vi "RFSG_Control.vi"(8 "error in (no error)":errorcluster, 10 "Device Resources":T1={"RFSG Resource in"="5646R", "RFSA Resource in"="5646R", "RFmx Resource in"=""}, 11 "Message_Queues":T2) -> (0 "error out":errorcluster)   [LabVIEW 2014]
uses:
  02_Controls/Message_Queues.ctl
  02_Controls/Message_Data_Ctl.ctl
  15_DataManagement/Device_Resources.ctl
  15_DataManagement/Config_RFSG.ctl
  <instrlib>/niRFSG/niRFSG.llb/niRFSG Signal Names.ctl
  <instrlib>/niRFSG/niRFSG.llb/niRFSG Signal Identifiers.ctl
  <instrlib>/niRFSG/niRFSG.llb/niRFSG Exported Signal Destinations.ctl
  15_DataManagement/Change_Parameters.ctl
  <vilib>/RF Toolkits/GSM-EDGE/niGSMEDGE.lvlib
panel:
  out "Message":string
  in  "WfmList":string[](array[string])=["LTE", "WCDMA", "GSM", "EDGE", "CW", "CWM"]
  out "RFSG Resource out":refnum<k15>="5644R (17)"
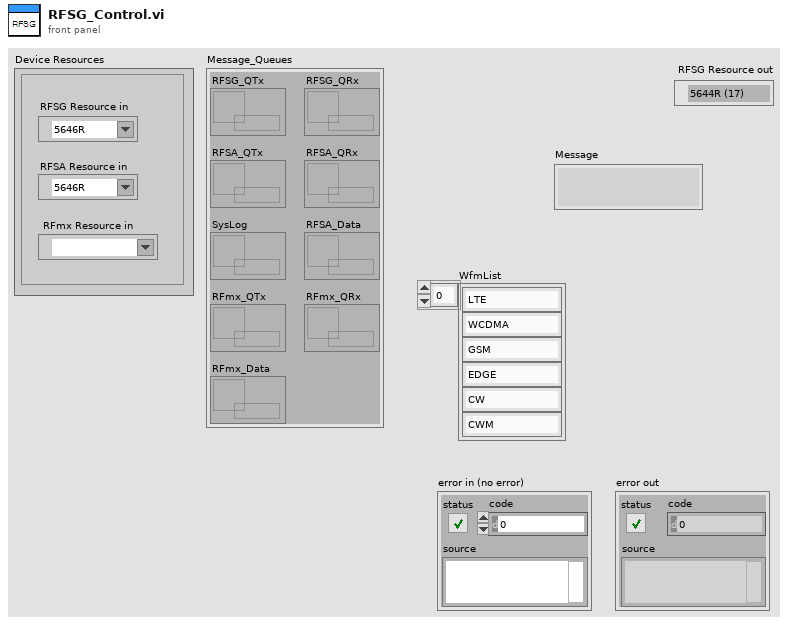
[diagram p1: front panel]
types:
  T1 = typedef "Device_Resources.ctl" = cluster{"RFSG Resource in":refnum<k15>, "RFSA Resource in":refnum<k15>, "RFmx Resource in":refnum<k15>}
  T2 = typedef "Message_Queues.ctl" = cluster{"RFSG_QTx":refnum<queue>, "RFSG_QRx":refnum<queue>, "RFSA_QTx":refnum<queue>, "RFSA_QRx":refnum<queue>, "SysLog":refnum<queue>, "RFSA_Data":refnum<queue>, "RFmx_QTx":refnum<queue>, "RFmx_QRx":refnum<queue>, "RFmx_Data":refnum<queue>}
  T3 = typedef "Config_RFSG.ctl" = cluster{"Carrier Frequency":dbl, "RF Power Level (dBm)":dbl, "SG External Gain (dBm)":dbl, "Standard":enum16{"LTE", "WCDMA", "GSM", "EDGE", "CW", "CWM"}}
  T4 = typedef "niRFSG Exported Signal Destinations.ctl" = string
  T5 = typedef "niRFSG Signal Identifiers.ctl" = string
  T6 = typedef "Change_Parameters.ctl" = cluster{"UpdateCmd":string, "Index":i32, "Carrier_Freq":dbl, "RF_Power":dbl, "Standard":enum16{"LTE", "WCDMA", "GSM", "EDGE", "CW"}, "Ref_Level_Offset":dbl}
  T7 = typedef "niRFSG Signal Names.ctl" = i32
  T8 = enum16{"LTE", "WCDMA", "GSM", "EDGE", "CW", "CWM"}
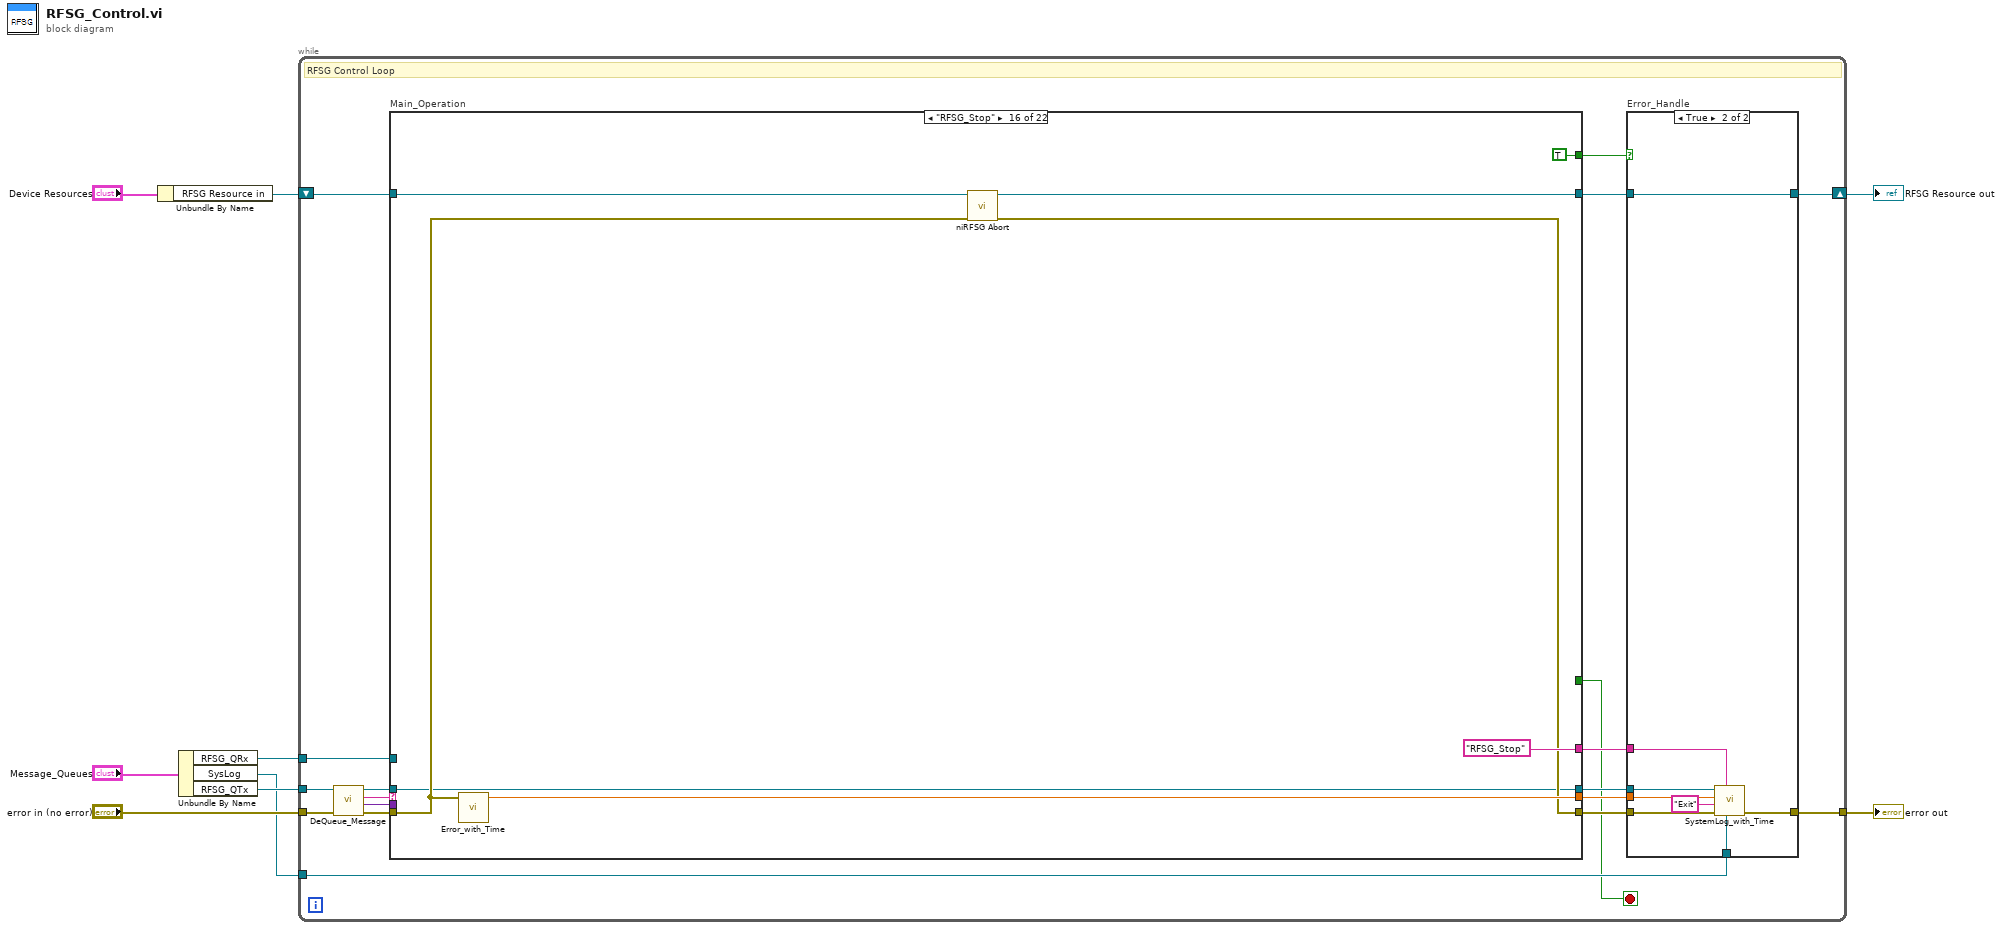
[diagram p0: block diagram]
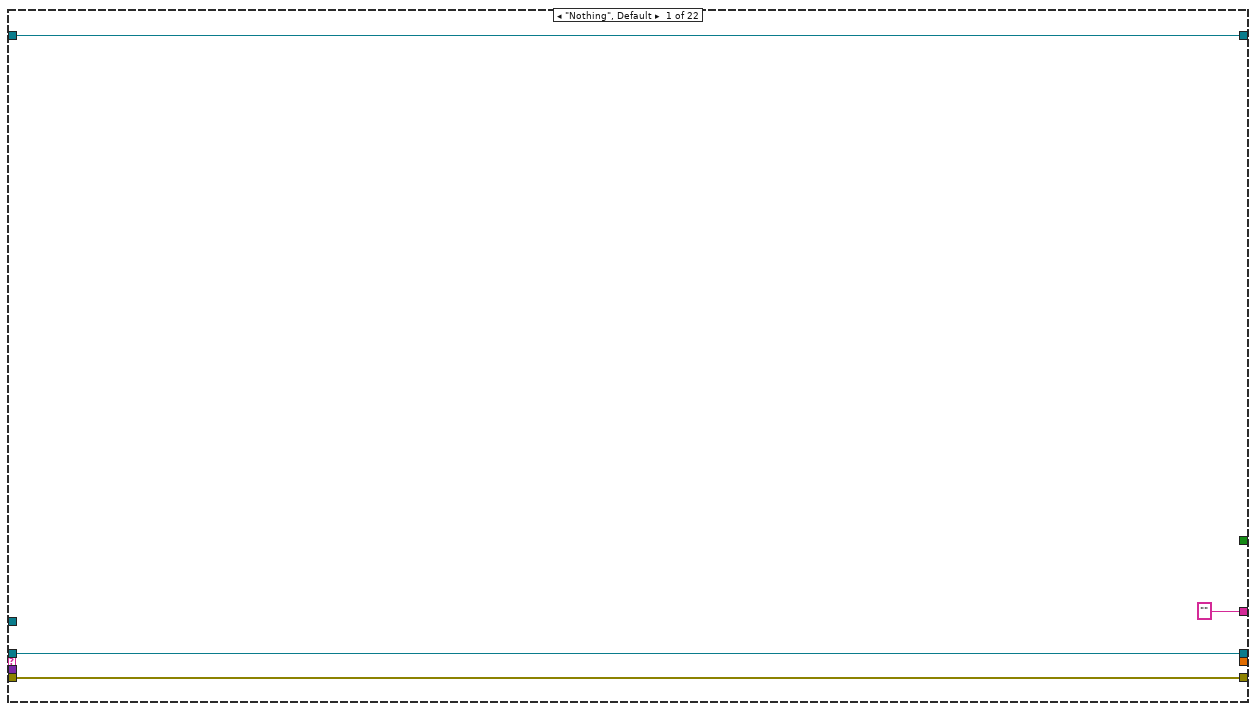
[diagram p3: hidden frame]
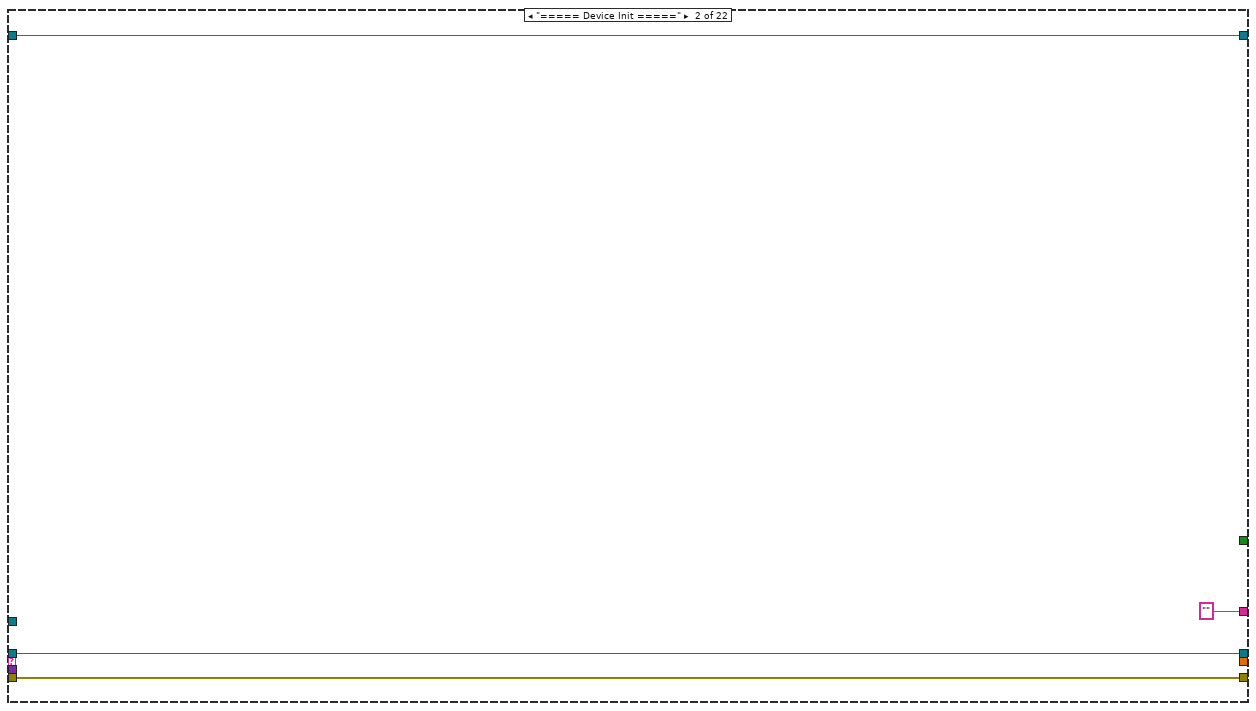
[diagram p4: hidden frame]
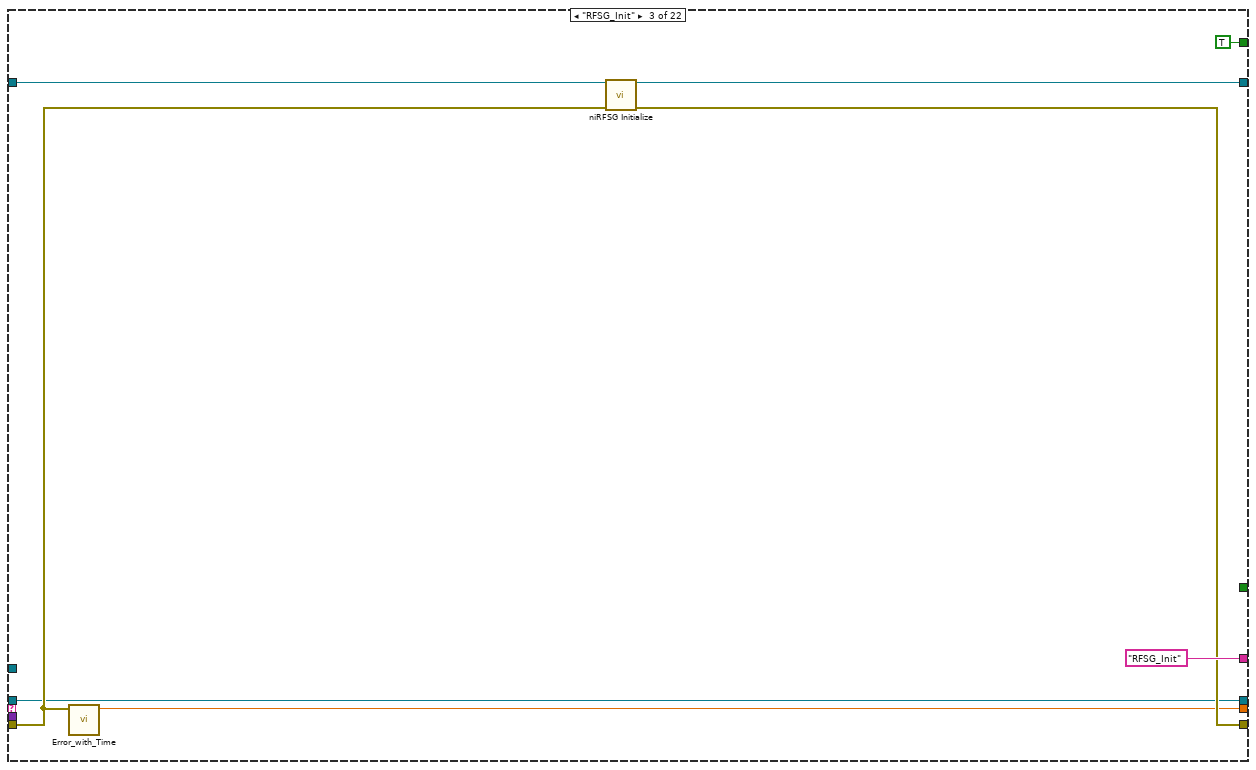
[diagram p5: hidden frame]
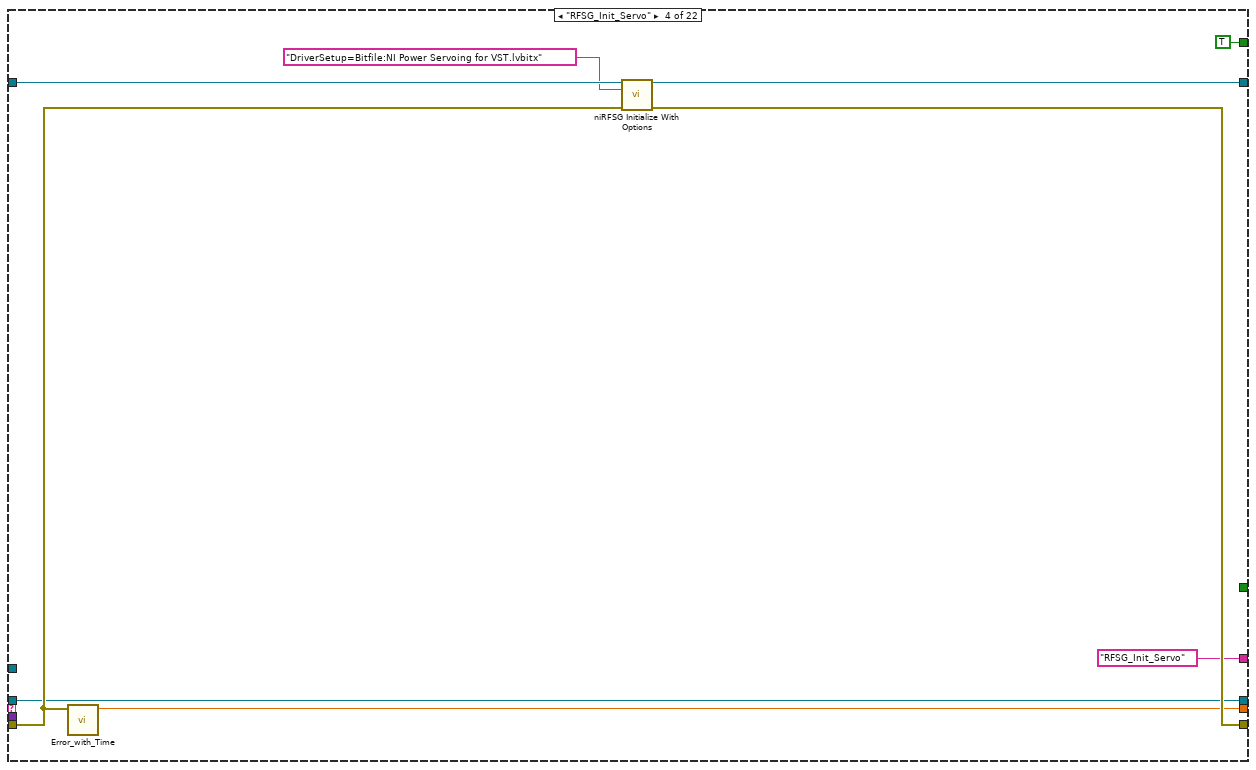
[diagram p6: hidden frame]
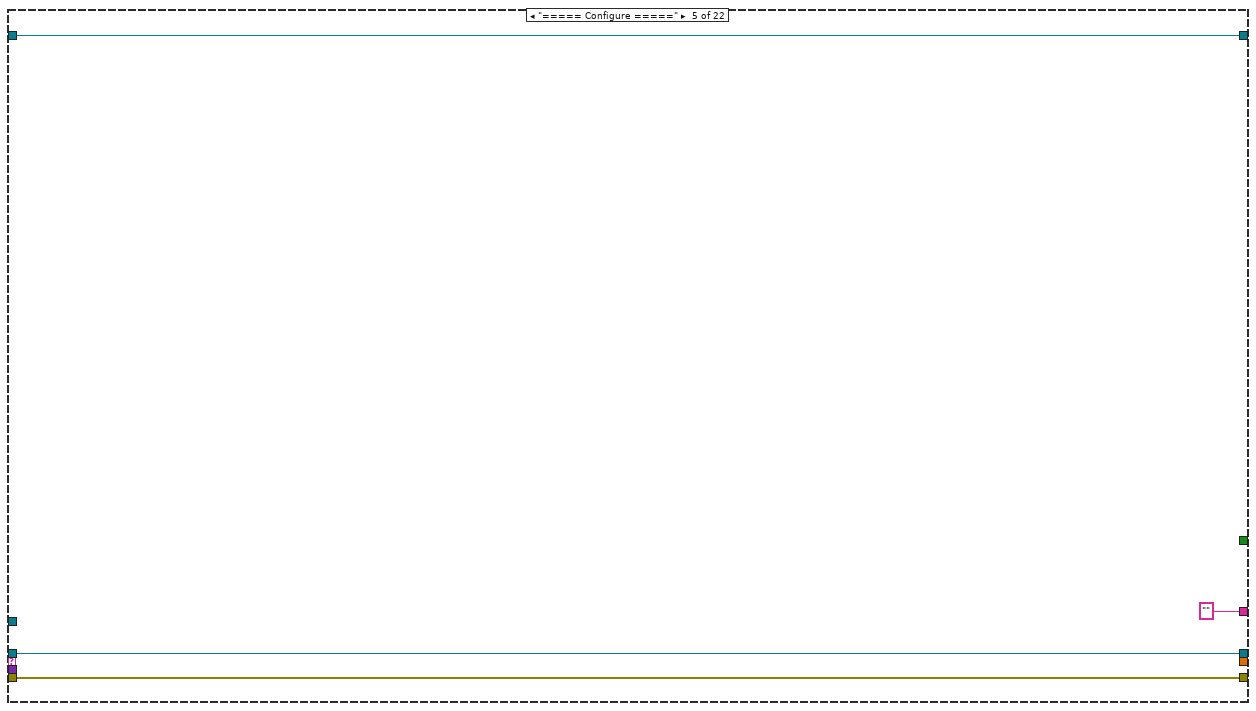
[diagram p7: hidden frame]
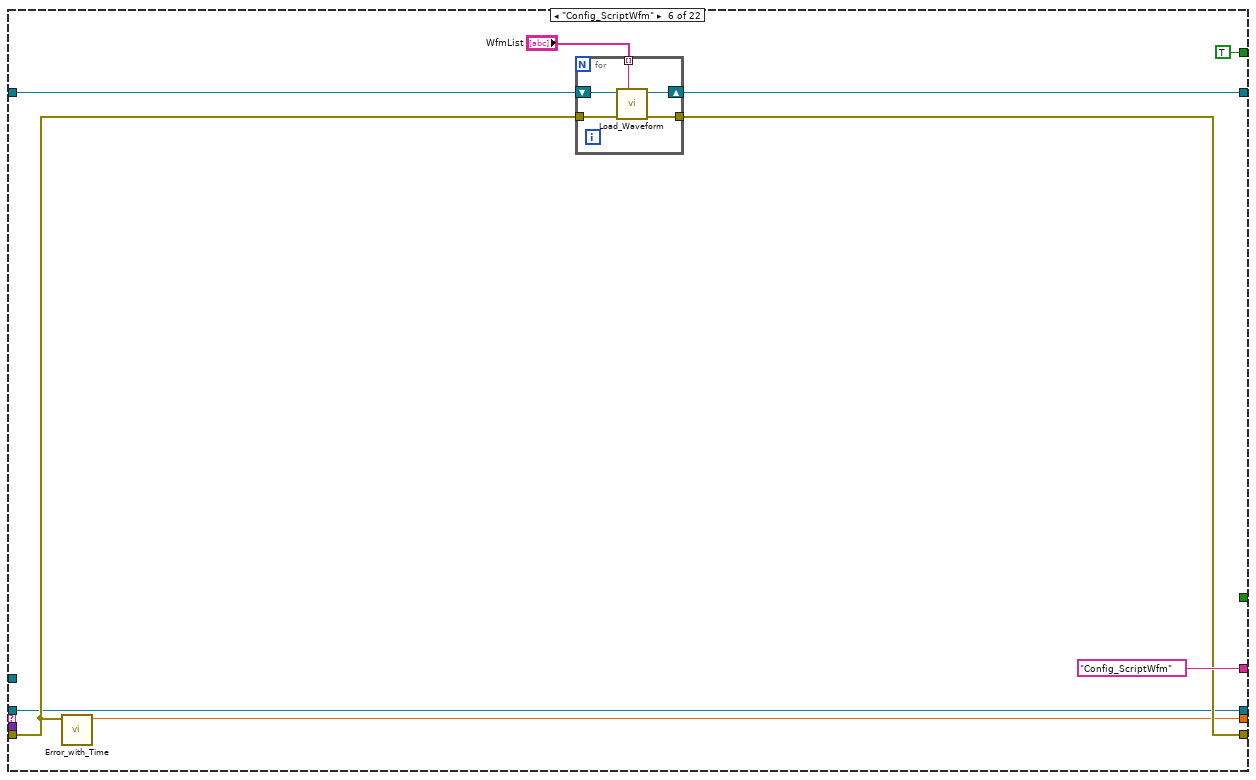
[diagram p8: hidden frame]
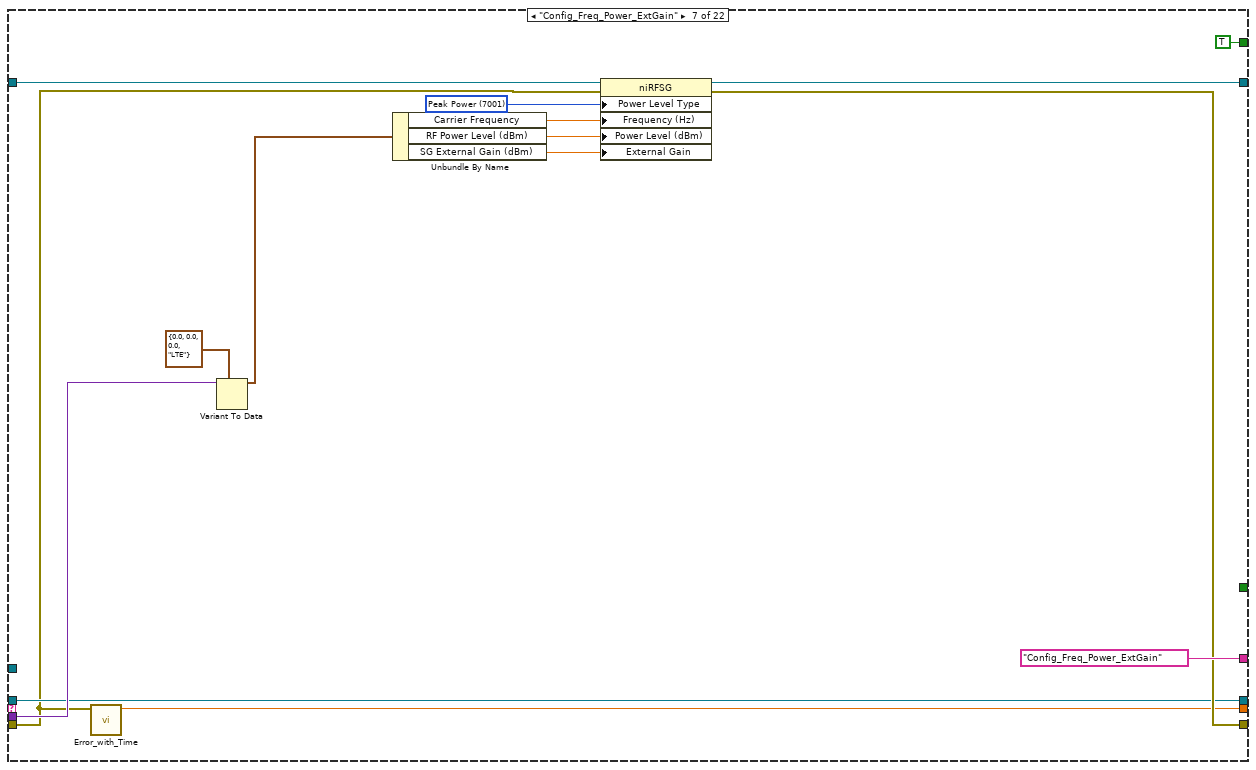
[diagram p9: hidden frame]
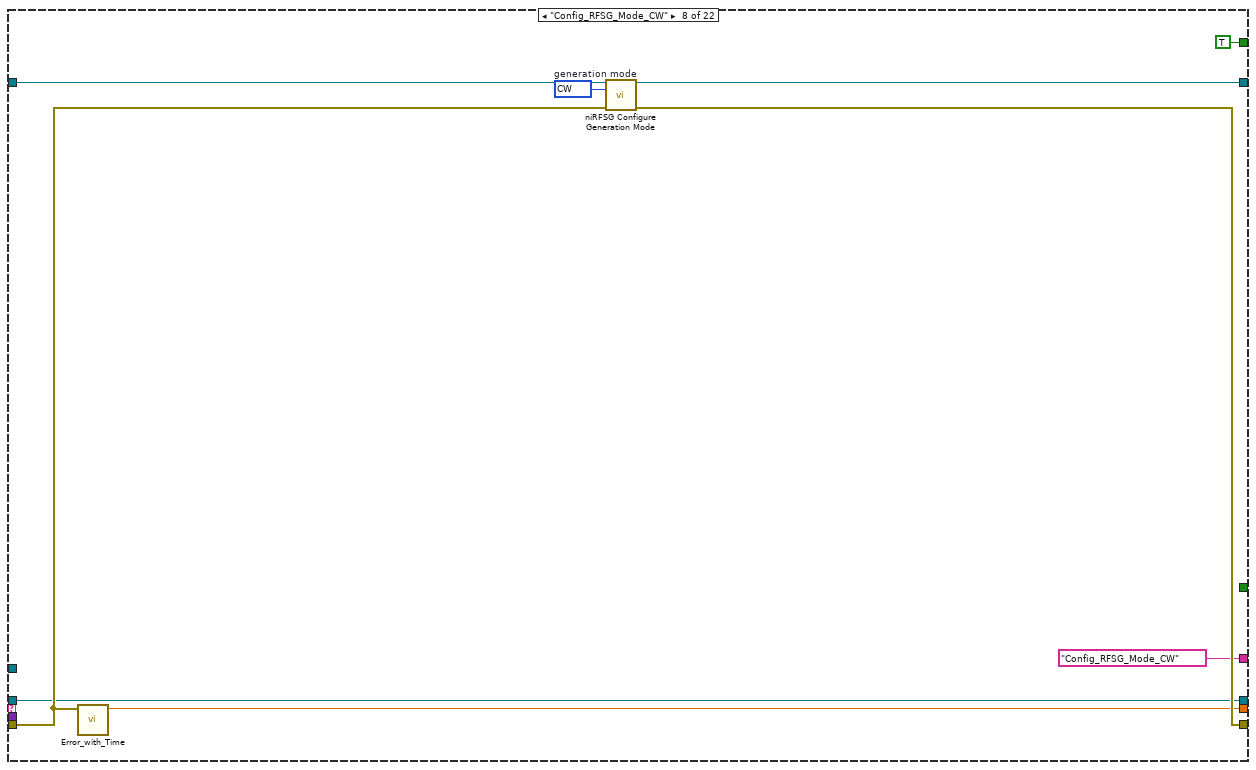
[diagram p10: hidden frame]
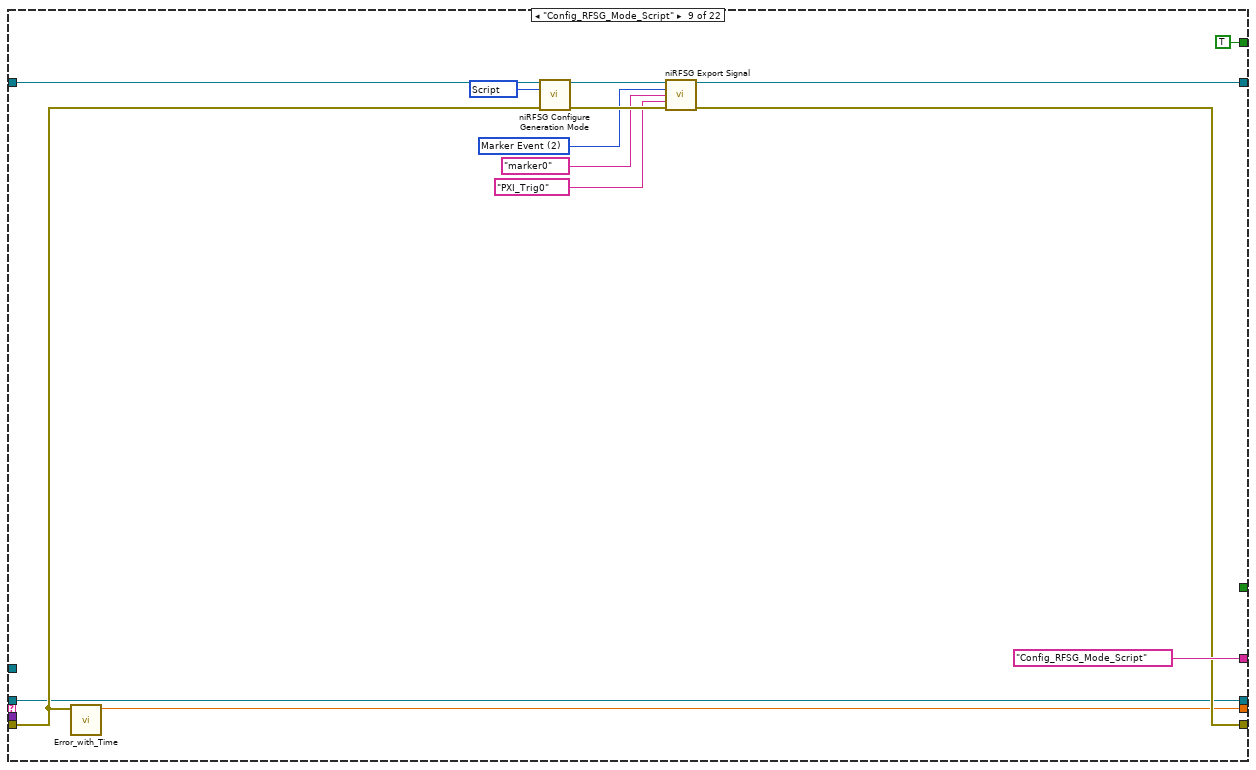
[diagram p11: hidden frame]
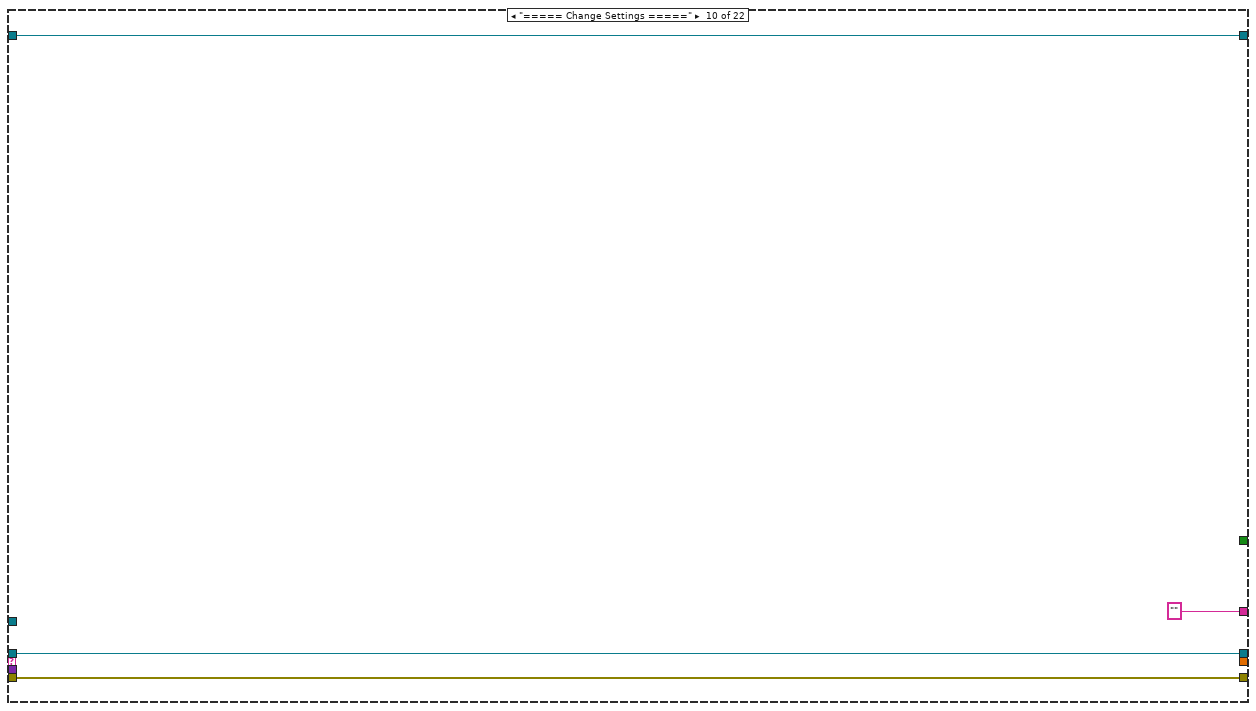
[diagram p12: hidden frame]
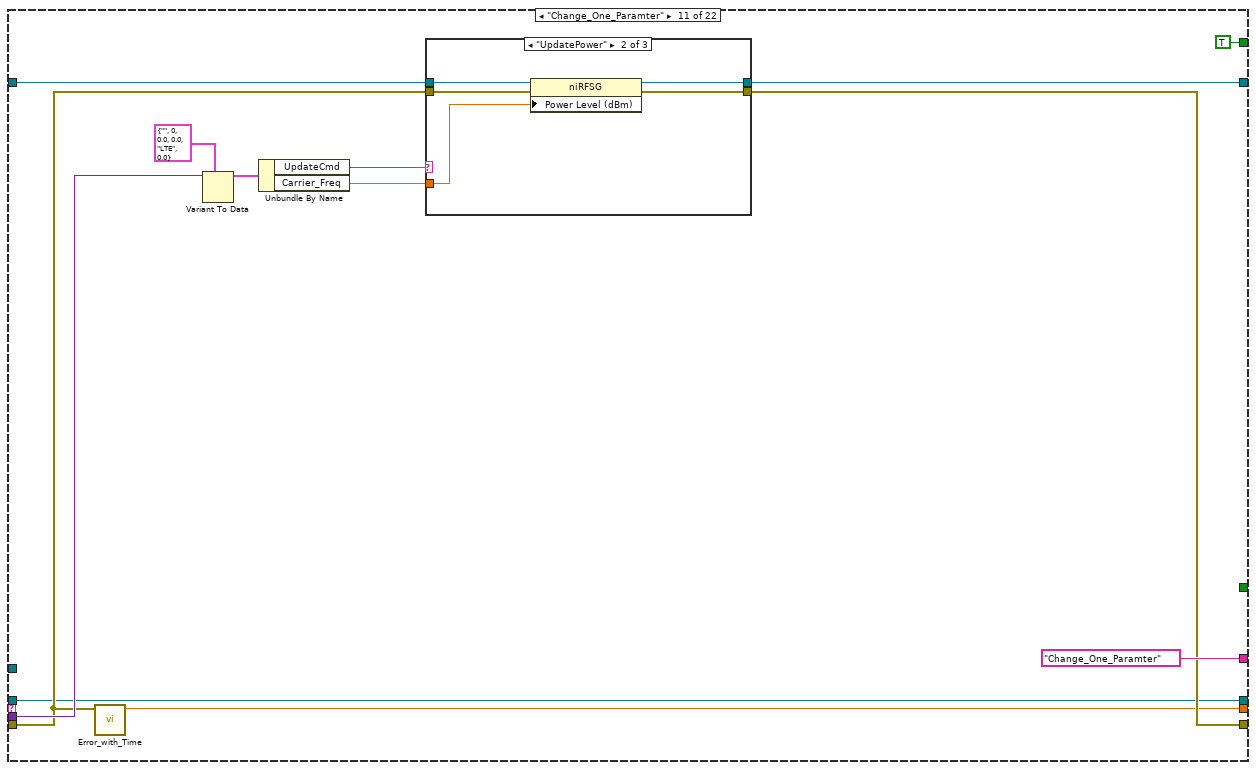
[diagram p13: hidden frame]
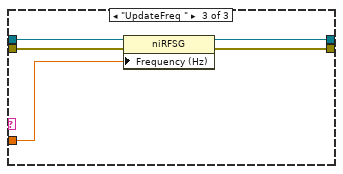
[diagram p15: hidden frame]
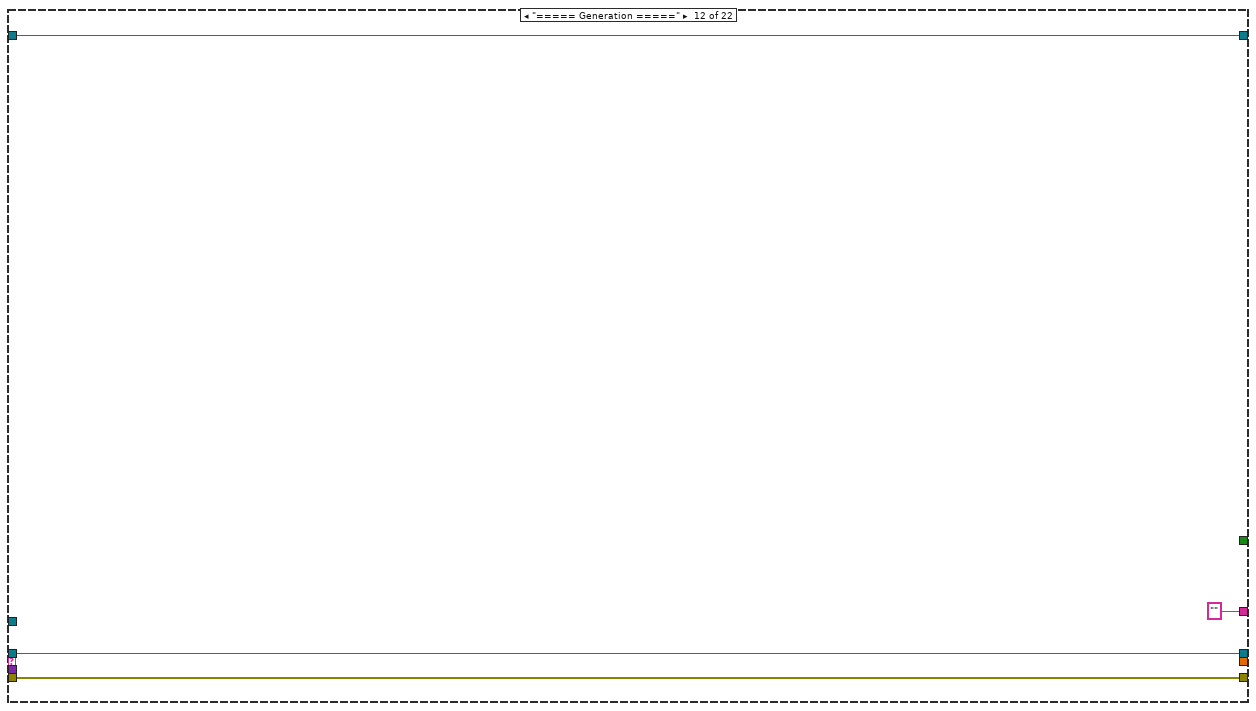
[diagram p16: hidden frame]
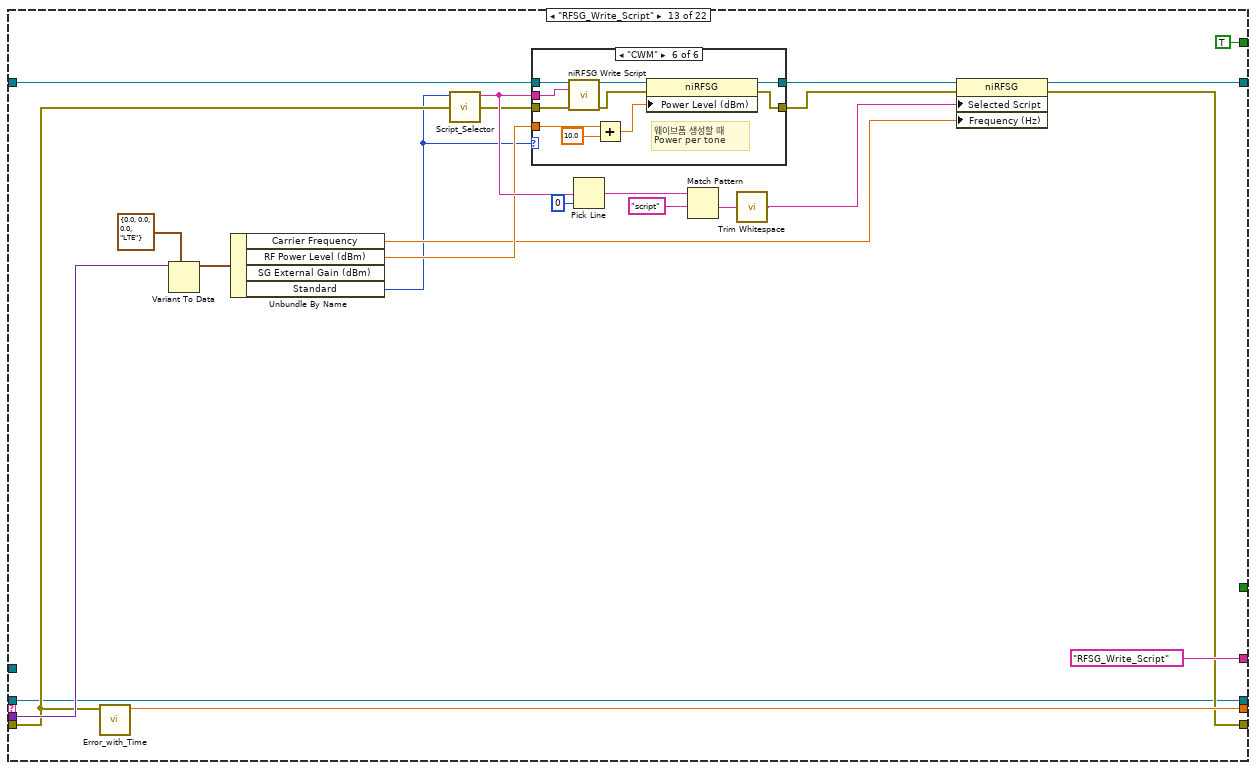
[diagram p17: hidden frame]
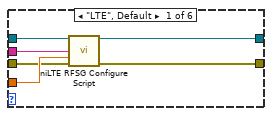
[diagram p18: hidden frame]
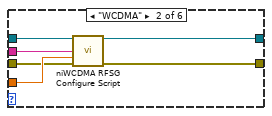
[diagram p19: hidden frame]
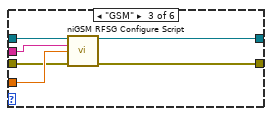
[diagram p20: hidden frame]
diagram:
  n1 = Unbundle By Name("Device Resources") -> ("RFSG Resource in"=w1:refnum<k15>)
  n2 = Unbundle By Name("Message_Queues") -> ("RFSG_QRx"=w4:refnum<queue>, "SysLog"=w3:refnum<queue>, "RFSG_QTx"=w7:refnum<queue>)
  n3 = while {
    tunnel: "error in (no error)" -> [w27]
    tunnel: [w19] -> w8
    tunnel: w7 -> [w22]
    shift-right: [w11] -> w5
    shift-left: w1 -> [w21]
    tunnel: w4 -> [w20]
    tunnel: w3 -> [w14]
    stop <- w13 stop-if-true
    # "RFSG Control Loop"
    n4 = call "DeQueue_Message.vi"("error in (no error)"=w27, "Message_Queue"=w22) -> ("error out"=w23:errorcluster, "Message Data"=w25:variant, "Message"=w26:string, "Dup_Message_Queue"=w24:refnum<queue>)  [unwired: 6 in]
    n5 = case "Main_Operation" shown="\"RFSG_Stop\"" w26 {
      tunnel: w25 -> [_ _ _ _ _ _ w93 _ _ _ w132 _ w172 _ _ _ _ _ _ _ _ _]
      tunnel: w24 -> [w38 w42 w47 w55 w63 w68 w83 w97 w106 w119 w124 w148 w153 w217 w224 w229 w237 w244 w252 _ _ w275]
      tunnel: w23 -> [w41 w45 w48 w56 w66 w69 w82 w98 w107 w121 w125 w151 w156 w219 w226 w232 w239 w246 w249 w257 w265 w272]
      tunnel: [_ _ _ _ _ _ _ _ _ _ _ _ _ _ _ _ _ _ _ _ _ TRUE] -> w13
      tunnel: [w41 w45 w50 w62 w66 w71 w85 w101 w109 w121 w127 w151 w154 w218 w226 w231 w243 w246 w254 w263 w271 w272] -> w17
      tunnel: w21 -> [w40 w44 w53 w61 w65 w74 w95 w103 w112 w122 w135 w150 w162 w223 w227 w230 w242 w247 w255 w261 w269 w277]
      tunnel: [w40 w44 w52 w60 w65 w73 w94 w102 w111 w122 w134 w150 w159 w222 w227 w235 refnum<k15> "5644R (17)" ("RFSG Resource out") w247 w255 w261 w269 w277] -> w12
      tunnel: w20 -> [_ _ _ _ _ _ _ _ _ _ _ _ _ _ _ _ _ _ _ w260 w268 _]
      tunnel: ["" ("Message") "" ("Message") "RFSG_Init" ("Message") "RFSG_Init_Servo" ("Message") "" ("Message") "Config_ScriptWfm" ("Message") "Config_Freq_Power_ExtGain" ("Message") "Config_RFSG_Mode_CW" ("Message") "Config_RFSG_Mode_Script" ("Message") "" ("Message") "Change_One_Paramter" ("Message") "" ("Message") "RFSG_Write_Script" ("Message") "RFSG_Initiate" ("Message") "" ("Message") "RFSG_Stop" ("Message") "RFSG_Close" ("Message") "" ("Message") "Wait_Cmd" ("Message") "Send_to_Cmd" ("Message") "Send_to_RFSA" ("Message") "RFSG_Exit" ("Message")] -> w18
      tunnel: [_ _ w49 w57 _ w70 w84 w99 w108 _ w126 _ w157 w220 _ w233 w240 _ w248 w256 w264 w273] -> w16
      tunnel: [w38 w42 w47 w55 w63 w68 w83 w97 w106 w119 w124 w148 w153 w217 w224 w229 w237 w244 w252 w260 w268 w275] -> w15
      tunnel: [_ _ TRUE TRUE _ TRUE TRUE TRUE TRUE _ TRUE _ TRUE TRUE _ TRUE TRUE _ TRUE TRUE TRUE TRUE] -> w10
      frame "Nothing", Default {
      }
      frame "===== Device Init =====" {
      }
      frame "RFSG_Init" {
        n6 = call "Error_with_Time.vi"("error in (no error)"=w48) -> ("relative seconds"=w49:dbl)  [unwired: 10 in]
        n7 = call <instrlib>:"niRFSG Initialize.vi"("resource name"=w53, "error in"=w48) -> ("instrument handle"=w52:refnum<k15>, "error out"=w50:errorcluster)  [unwired: 12 in]
      }
      frame "RFSG_Init_Servo" {
        n8 = call "Error_with_Time.vi"("error in (no error)"=w56) -> ("relative seconds"=w57:dbl)  [unwired: 10 in]
        n9 = call <instrlib>:"niRFSG Initialize With Options.vi"("resource name"=w61, "option string"="DriverSetup=Bitfile:NI Power Servoing for VST.lvbitx" ("Bitfile"), "error in"=w56) -> ("instrument handle"=w60:refnum<k15>, "error out"=w62:errorcluster)  [unwired: 11 in]
      }
      frame "===== Configure =====" {
      }
      frame "Config_ScriptWfm" {
        n10 = call "Error_with_Time.vi"("error in (no error)"=w69) -> ("relative seconds"=w70:dbl)  [unwired: 10 in]
        n11 = for {
          shift-right: [w79] -> w73
          shift-left: w74 -> [w80]
          tunnel: "WfmList" -> [w78] mode=indexing
          tunnel: w69 -> [w77]
          tunnel: [w76] -> w71
          n12 = call "Load_Waveform.vi"("Cmd"=w78, "error in"=w77, "RFSG_In"=w80) -> ("error out"=w76:errorcluster, "RFSG_Out"=w79:refnum<k15>)  [unwired: 7 in]
        }
      }
      frame "Config_Freq_Power_ExtGain" {
        w87 = 7001 items=["Average Power"=7000, "Peak Power"=7001] ("RF:Power Level Type")
        n13 = call "Error_with_Time.vi"("error in (no error)"=w82) -> ("relative seconds"=w84:dbl)  [unwired: 10 in]
        n14 = Variant To Data(type=T3 {"Carrier Frequency"=0.0, "RF Power Level (dBm)"=0.0, "SG External Gain (dBm)"=0.0, "Standard"=enum."LTE"} ("RFSG_Config"), Variant=w93) -> (data=w91:T3)  [unwired: 1 in, 1 out]
        n15 = Unbundle By Name(w91) -> ("Carrier Frequency"=w88:dbl, "RF Power Level (dBm)"=w90:dbl, "SG External Gain (dBm)"=w89:dbl)
        n16 = property class="niRFSG"(reference=w95, error in=w82, "Power Level Type"=w87, "Frequency (Hz)"=w88, "Power Level (dBm)"=w90, "External Gain"=w89) -> (reference out=w94:refnum<k15>, error out=w85:errorcluster)
      }
      frame "Config_RFSG_Mode_CW" {
        w104 = 1000 items=["CW"=1000, "Arb Waveform"=1001, "Script"=1002]  # generation mode
        n17 = call "Error_with_Time.vi"("error in (no error)"=w98) -> ("relative seconds"=w99:dbl)  [unwired: 10 in]
        n18 = call <instrlib>:"niRFSG Configure Generation Mode.vi"("instrument handle"=w103, "generation mode"=w104, "error in"=w98) -> ("instrument handle out"=w102:refnum<k15>, "error out"=w101:errorcluster)  [unwired: 11 in]
      }
      frame "Config_RFSG_Mode_Script" {
        w113 = T7 2 items=["Start Trigger", "Script Trigger", "Marker Event", "Ref Clock", "Started Event", "Done Event", "Configuration List Step Trigger"] ("signal")
        w118 = 1002 items=["CW"=1000, "Arb Waveform"=1001, "Script"=1002] ("generation mode")
        n19 = call "Error_with_Time.vi"("error in (no error)"=w107) -> ("relative seconds"=w108:dbl)  [unwired: 10 in]
        n20 = call <instrlib>:"niRFSG Configure Generation Mode.vi"("instrument handle"=w112, "generation mode"=w118, "error in"=w107) -> ("instrument handle out"=w117:refnum<k15>, "error out"=w116:errorcluster)  [unwired: 11 in]
        n21 = call <instrlib>:"niRFSG Export Signal.vi"("instrument handle"=w117, "signal"=w113, "signal identifier"=T5 "marker0", "output terminal"=T4 "PXI_Trig0", "error in"=w116) -> ("instrument handle out"=w111:refnum<k15>, "error out"=w109:errorcluster)  [unwired: 9 in]
      }
      frame "===== Change Settings =====" {
      }
      frame "Change_One_Paramter" {
        n22 = call "Error_with_Time.vi"("error in (no error)"=w125) -> ("relative seconds"=w126:dbl)  [unwired: 10 in]
        n23 = Variant To Data(type=T6 {"UpdateCmd"="", "Index"=0, "Carrier_Freq"=0.0, "RF_Power"=0.0, "Standard"=enum."LTE", "Ref_Level_Offset"=0.0} ("Change_RFSG_one_Parameter"), Variant=w132) -> (data=w131:T6)  [unwired: 1 in, 1 out]
        n24 = Unbundle By Name(w131) -> ("UpdateCmd"=w130:string, "Carrier_Freq"=w129:dbl)
        n25 = case shown="\"UpdatePower\"" w130 {
          tunnel: w135 -> [w137 w142 w147]
          tunnel: [w137 w141 w146] -> w134
          tunnel: w129 -> [_ w140 w145]
          tunnel: w125 -> [w136 w139 w144]
          tunnel: [w136 w138 w143] -> w127
          frame "Nothing", Default {
          }
          frame "UpdatePower" {
            n26 = property class="niRFSG"(reference=w142, error in=w139, "Power Level (dBm)"=w140) -> (reference out=w141:refnum<k15>, error out=w138:errorcluster)
          }
          frame "UpdateFreq " {
            n27 = property class="niRFSG"(reference=w147, error in=w144, "Frequency (Hz)"=w145) -> (reference out=w146:refnum<k15>, error out=w143:errorcluster)
          }
        }
      }
      frame "===== Generation =====" {
      }
      frame "RFSG_Write_Script" {
        n28 = call "Error_with_Time.vi"("error in (no error)"=w156) -> ("relative seconds"=w157:dbl)  [unwired: 10 in]
        n29 = Variant To Data(type=T3 {"Carrier Frequency"=0.0, "RF Power Level (dBm)"=0.0, "SG External Gain (dBm)"=0.0, "Standard"=enum."LTE"} ("RFSG_Config"), Variant=w172) -> (data=w171:T3)  [unwired: 1 in, 1 out]
        n30 = Unbundle By Name(w171) -> ("Carrier Frequency"=w160:dbl, "RF Power Level (dBm)"=w161:dbl, "Standard"=w155:T8)  [unwired: 1 out]
        n31 = call "Script_Selector.vi"("Standard"=w155) -> ("Script"=w163:string)  [unwired: 10 in]
        n32 = case shown="\"CWM\"" w155 {
          tunnel: w162 -> [w179 w185 w191 w197 w205 w215]
          tunnel: [w178 w184 w190 w196 w199 w210] -> w170
          tunnel: w163 -> [w177 w183 w189 w195 w203 w213]
          tunnel: w161 -> [w176 w182 w188 w194 w200 w208]
          tunnel: w156 -> [w175 w181 w187 w193 w204 w214]
          tunnel: [w174 w180 w186 w192 w198 w209] -> w169
          frame "LTE", Default {
            n33 = call <vilib>:"niLTE RFSG Configure Script.vi"("instrument handle"=w179, "script"=w177, "power level (dBm)"=w176, "error in"=w175) -> ("instrument handle out"=w178:refnum<k15>, "error out"=w174:errorcluster)  [unwired: 10 in]
          }
          frame "WCDMA" {
            n34 = call <vilib>:"niWCDMA RFSG Configure Script.vi"("instrument handle"=w185, "script"=w183, "power level (dBm)"=w182, "error in"=w181) -> ("instrument handle out"=w184:refnum<k15>, "error out"=w180:errorcluster)  [unwired: 10 in]
          }
          frame "GSM" {
            n35 = call <vilib>:"niGSM RFSG Configure Script.vi"("instrument handle in"=w191, "script"=w189, "power level (dBm)"=w188, "error in"=w187) -> ("instrument handle out"=w190:refnum<k15>, "error out"=w186:errorcluster)  [unwired: 10 in]
          }
          frame "EDGE" {
            n36 = call <vilib>:"niEDGE RFSG Configure Script.vi"("instrument handle in"=w197, "script"=w195, "power level (dBm)"=w194, "error in"=w193) -> ("instrument handle out"=w196:refnum<k15>, "error out"=w192:errorcluster)  [unwired: 10 in]
          }
          frame "CW" {
            n37 = call <instrlib>:"niRFSG Write Script.vi"("instrument handle"=w205, "script"=w203, "error in"=w204) -> ("instrument handle out"=w202:refnum<k15>, "error out"=w201:errorcluster)  [unwired: 11 in]
            n38 = property class="niRFSG"(reference=w202, error in=w201, "Power Level (dBm)"=w200) -> (reference out=w199:refnum<k15>, error out=w198:errorcluster)
          }
          frame "CWM" {
            # "웨이브폼 생성할 때\nPower per tone"
            n39 = call <instrlib>:"niRFSG Write Script.vi"("instrument handle"=w215, "script"=w213, "error in"=w214) -> ("instrument handle out"=w212:refnum<k15>, "error out"=w211:errorcluster)  [unwired: 11 in]
            n40 = Add(x=w208, y=10.0) -> (x+y=w206:dbl)
            n41 = property class="niRFSG"(reference=w212, error in=w211, "Power Level (dBm)"=w206) -> (reference out=w210:refnum<k15>, error out=w209:errorcluster)
          }
        }
        n42 = Pick Line(multi-line string=w163, line index=0) -> (output string=w166:string)  [unwired: 1 out]
        n43 = Match Pattern(string=w166, regular expression="script") -> (after substring=w165:string)  [unwired: 4 out]
        n44 = call <vilib>:"Trim Whitespace.vi"("string"=w165) -> ("trimmed string"=w164:string)  [unwired: 1 in]
        n45 = property class="niRFSG"(reference=w170, error in=w169, "Selected Script"=w164, "Frequency (Hz)"=w160) -> (reference out=w159:refnum<k15>, error out=w154:errorcluster)
      }
      frame "RFSG_Initiate" {
        n46 = call "Error_with_Time.vi"("error in (no error)"=w219) -> ("relative seconds"=w220:dbl)  [unwired: 10 in]
        n47 = call <instrlib>:"niRFSG Initiate.vi"("instrument handle"=w223, "error in"=w219) -> ("instrument handle out"=w222:refnum<k15>, "error out"=w218:errorcluster)  [unwired: 12 in]
      }
      frame "===== Session Stop&Close =====" {
      }
      frame "RFSG_Stop" {
        n48 = call "Error_with_Time.vi"("error in (no error)"=w232) -> ("relative seconds"=w233:dbl)  [unwired: 10 in]
        n49 = call <instrlib>:"niRFSG Abort.vi"("instrument handle"=w230, "error in"=w232) -> ("instrument handle out"=w235:refnum<k15>, "error out"=w231:errorcluster)  [unwired: 12 in]
      }
      frame "RFSG_Close" {
        n50 = call "Error_with_Time.vi"("error in (no error)"=w239) -> ("relative seconds"=w240:dbl)  [unwired: 10 in]
        n51 = call <instrlib>:"niRFSG Close.vi"("instrument handle"=w242, "error in"=w239) -> ("error out"=w243:errorcluster)  [unwired: 13 in]
      }
      frame "===== Operation =====" {
      }
      frame "Wait_Cmd" {
        n52 = call "Error_with_Time.vi"("error in (no error)"=w249) -> ("relative seconds"=w248:dbl)  [unwired: 10 in]
        n53 = call "DeQueue_Message.vi"("error in (no error)"=w249, "Message_Queue"=w252) -> ("error out"=w254:errorcluster, "Message"=→"Message":string)  [unwired: 6 in, 2 out]
      }
      frame "Send_to_Cmd" {
        n54 = call "Error_with_Time.vi"("error in (no error)"=w257) -> ("relative seconds"=w256:dbl)  [unwired: 10 in]
        n55 = call "EnQueue_Message_Single.vi"("error in (no error)"=w257, "Message"="OK", "Message_Queue"=w260) -> ("error out"=w263:errorcluster)  [unwired: 7 in, 1 out]
      }
      frame "Send_to_RFSA" {
        n56 = call "Error_with_Time.vi"("error in (no error)"=w265) -> ("relative seconds"=w264:dbl)  [unwired: 10 in]
        n57 = call "EnQueue_Message_Single.vi"("error in (no error)"=w265, "Message"="RFSG_Initiated", "Message_Queue"=w268) -> ("error out"=w271:errorcluster)  [unwired: 7 in, 1 out]
      }
      frame "Exit" {
        n58 = call "Error_with_Time.vi"("error in (no error)"=w272) -> ("relative seconds"=w273:dbl)  [unwired: 10 in]
      }
    }
    n59 = case "Error_Handle" shown="True" w10 {
      tunnel: w17 -> [w29 w37]
      tunnel: [w29 w36] -> w19
      tunnel: w18 -> [_ w35]
      tunnel: w15 -> [_ w34]
      tunnel: w16 -> [_ w33]
      tunnel: w14 -> [_ w32]
      tunnel: w12 -> [w28 w30]
      tunnel: [w28 w30] -> w11
      frame False {
      }
      frame True {
        n60 = call "SystemLog_with_Time.vi"("SysLog_Queue"=w32, "Message_in"=w35, "error in (no error)"=w37, "Send_Msg"="Exit", "Tick_in"=w33, "Worker_Queue"=w34) -> ("error out"=w36:errorcluster)  [unwired: 5 in]
      }
    }
  }
  "error out" <- w8
  "RFSG Resource out" <- w5
